vi "Command List.vi"() -> (2 "TCP commands":string[](array[string]))   [LabVIEW 2021, in "AudioGenManageConnectionProcess.lvlib"]
uses:
  AudioGenManageConnectionProcess.lvlib
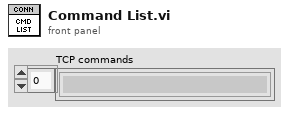
[diagram p1: front panel]
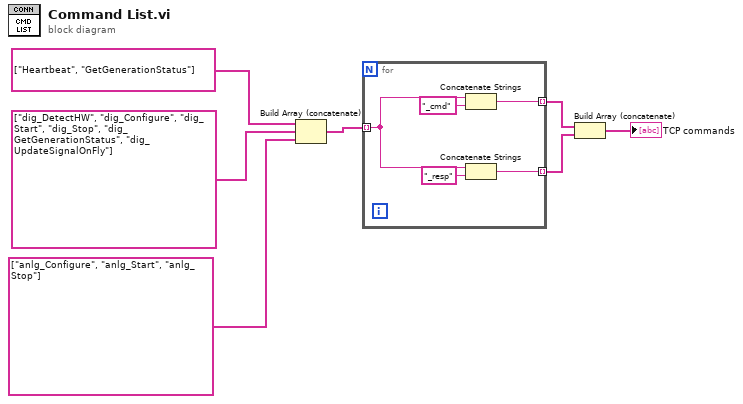
[diagram p0: block diagram]
diagram:
  n1 = Build Array (concatenate)(string[] ["Heartbeat", "GetGenerationStatus"], string[] ["dig_DetectHW", "dig_Configure", "dig_Start", "dig_Stop", "dig_GetGenerationStatus", "dig_UpdateSignalOnFly"], string[] ["anlg_Configure", "anlg_Start", "anlg_Stop"]) -> (w5:string[])
  n2 = for {
    tunnel: w5 -> [w12] mode=indexing
    tunnel: [w11] -> w4 mode=indexing
    tunnel: [w10] -> w3 mode=indexing
    n3 = Concatenate Strings(w12, "_cmd" ("string")) -> (w11:string)
    n4 = Concatenate Strings(w12, "_resp" ("string")) -> (w10:string)
  }
  n5 = Build Array (concatenate)(w4, w3) -> (→"TCP commands":string[])
